vi "ToplevelRunTest.vi"() -> ()   [LabVIEW 2014]
panel:
  in  "StartTest":bool
  in  "COM Port MicroZed":refnum<visa-resource-name>="COM4"
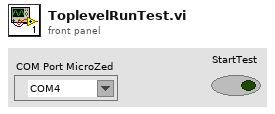
[diagram p1: front panel]
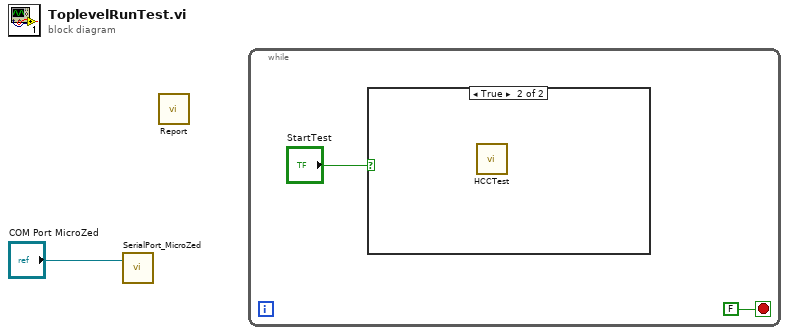
[diagram p0: block diagram]
diagram:
  n1 = call "SerialPort_MicroZed.vi"("COM Port"="COM Port MicroZed") -> ()  [unwired: 2 in, 1 out]
  n2 = call "Report.vi"() -> ()  [unwired: 12 in]
  n3 = while {
    stop <- FALSE stop-if-true
    n4 = case shown="True" "StartTest" {
      frame False {
      }
      frame True {
        n5 = call "HCCTest.vi"() -> ()  [unwired: 12 in]
      }
    }
  }
